vi "ReadMemoryNode.vi"(8 "Error In":errorcluster, 11 "Multiplexer Node In":refnum<k20>) -> (0 "Error Out":errorcluster, 2 "Memory":string[](array[string]), 3 "Multiplexer Node Out":refnum<k20>)   [LabVIEW 2012]
uses:
  <vilib>/xml/NI_XML.lvlib
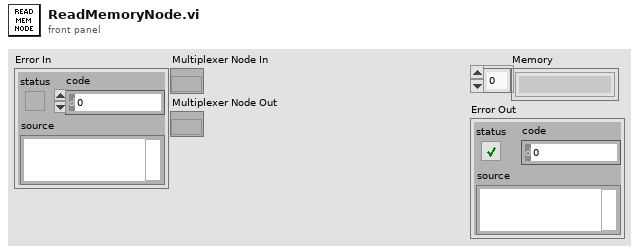
[diagram p1: front panel]
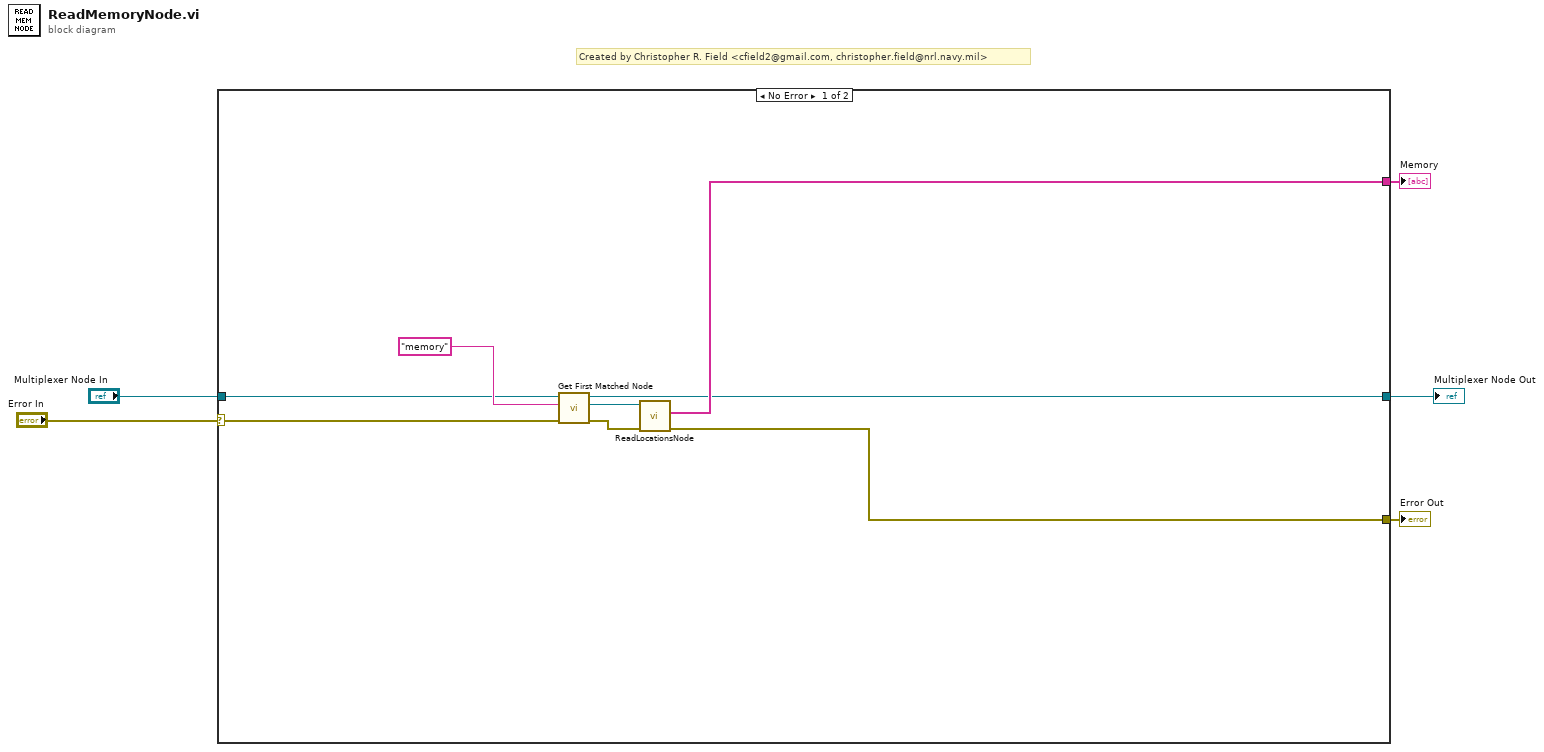
[diagram p0: block diagram]
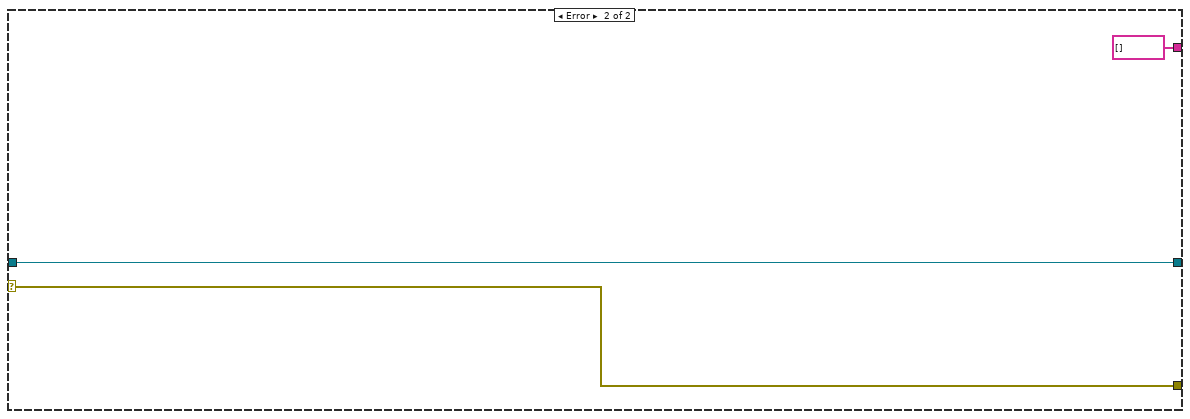
[diagram p2: hidden frame]
diagram:
  # "Created by Christopher R. Field <cfield2@gmail.com, christopher.field@nrl.navy.mil>"
  n1 = case shown="No Error" "Error In" {
    selector: "Error In" -> [w9 w16]
    tunnel: [w10 string[] [] ("Locations")] -> w5
    tunnel: "Multiplexer Node In" -> [w8 w15]
    tunnel: [w7 w15] -> w2
    tunnel: [w6 w16] -> w1
    frame No Error {
      n2 = call <vilib>:"Get First Matched Node.vi"("error in (no error)"=w9, "XPath expression"="memory", "node in"=w8) -> ("error out"=w11:errorcluster, "node result"=w12:refnum<k20>, "node out"=w7:refnum<k20>)  [unwired: 6 in]
      n3 = call "ReadLocationsNode.vi"("Error In"=w11, "Memory Node In"=w12) -> ("Error Out"=w6:errorcluster, "Locations"=w10:string[])  [unwired: 7 in, 1 out]
    }
    frame Error {
    }
  }
  "Memory" <- w5
  "Multiplexer Node Out" <- w2
  "Error Out" <- w1
